vi "Read.vi"(11 "ConfigMonitorInfoValue in":refnum<class "ConfigMonitorInfoValue.lvclass">) -> (2 "Info":T1[](array[typedef]))   [LabVIEW 2020, in "Volatus.lvlib" / "ConfigMonitorInfoValue.lvclass"]
uses:
  ConfigMonitorInfoValue.lvclass
  ConfigMonitorInfoValue.lvclass/ConfigMonitorInfoValue.ctl
  Config Alert Module/Node Config Info.ctl
  Volatus.lvlib
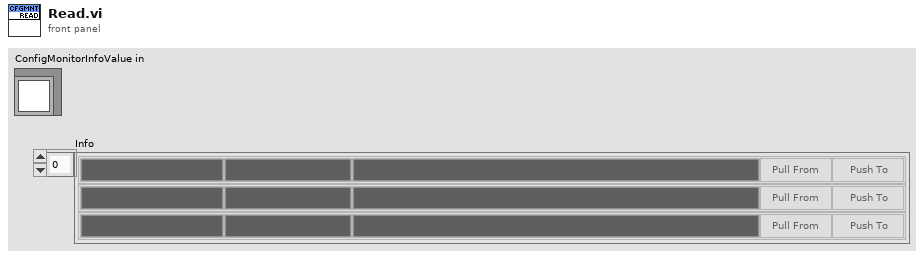
[diagram p1: front panel]
types:
  T1 = typedef "Volatus.lvlib/Node Config Info.ctl" = cluster{"Node":string, "Config Version":string, "Config Hash":string, "Pull":bool, "Push":bool, "Version Color":u32, "Hash Color":u32, "Node Color":u32}
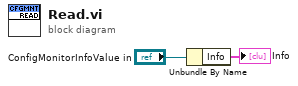
[diagram p0: block diagram]
diagram:
  n1 = Unbundle By Name("ConfigMonitorInfoValue in") -> ("Info"=→"Info":T1[])
